vi "Load by Identifier.vi"(8 "error in (no error)":errorcluster, 10 "Identifier":string, 11 "User Provider in":refnum<class "User Provider.lvclass">) -> (0 "error out":errorcluster, 2 "User":refnum<class "User.lvclass">, 3 "User Provider out":refnum<class "User Provider.lvclass">)   [LabVIEW 2022 SP3, in "HTTP-Conditum.lvlib" / "User Provider.lvclass"]
uses:
  User Provider.lvclass
  <vilib>/IlluminatedG/IG HTTP Server/HTTP Server/User/User.lvclass
  User Provider.lvclass/User Provider.ctl
  User/User.lvclass
  <vilib>/IlluminatedG/IG Conditum/Conditum/Columns/String/String.lvclass
  <vilib>/IlluminatedG/IG Conditum/Conditum/Entity Manager/Entity Manager.lvclass
  C:/Program Files (x86)/National Instruments/LabVIEW 2022/vi.lib/IlluminatedG/IG Conditum/Conditum/Entity/Entity.lvclass
  C:/Program Files (x86)/National Instruments/LabVIEW 2022/vi.lib/IlluminatedG/IG HTTP Server/HTTP Server/User/User.lvclass
  C:/Program Files (x86)/National Instruments/LabVIEW 2022/vi.lib/IlluminatedG/IG HTTP Server/HTTP Server/Service/Service.lvclass
  C:/dev/lv/illuminated-g/lv-http-conditum/HTTP-Conditum/User/User.lvclass
  C:/Program Files (x86)/National Instruments/LabVIEW 2022/vi.lib/IlluminatedG/IG Conditum/Conditum/Columns/Type/Type.lvclass
  C:/Program Files (x86)/National Instruments/LabVIEW 2022/vi.lib/IlluminatedG/IG Conditum/Conditum/Columns/String/String.lvclass
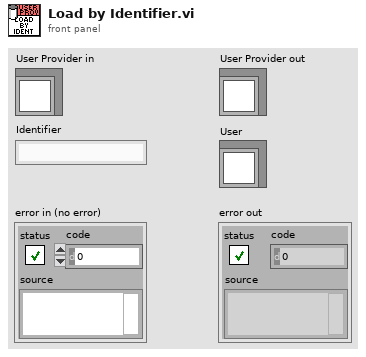
[diagram p1: front panel]
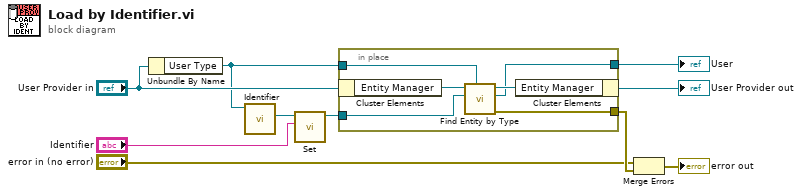
[diagram p0: block diagram]
diagram:
  n1 = Unbundle By Name("User Provider in") -> ("User Type"=w6:refnum<class "User.lvclass">)
  n2 = call "Identifier.vi"("User in"=w6) -> ("Identifier"=w10:refnum<class "String.lvclass">)  [unwired: 10 in]
  n3 = call <vilib>:"Set.vi"("Value"="Identifier", "String in"=w10) -> ("String out"=w8:refnum<class "String.lvclass">)  [unwired: 9 in]
  n4 = in-place {
    in-place-border: w8 -> [w15]
    in-place-border: w6 -> [w14]
    in-place-border: [w12] -> w5
    in-place-border: [w11] -> w3
    n5 = in-place-cluster #1("User Provider in") -> ("Entity Manager"=w16:refnum<class "Entity Manager.lvclass">)
    n6 = call <vilib>:"Find Entity by Type.vi"("Entity Type"=w14, "Type"=w15, "Entity Manager in"=w16) -> ("error out"=w11:errorcluster, "Entity"=w12:refnum<class "User.lvclass">, "Entity Manager out"=w13:refnum<class "Entity Manager.lvclass">)  [unwired: 6 in]
    n7 = in-place-cluster #1("Entity Manager"=w13) -> (→"User Provider out":refnum<class "User Provider.lvclass">)
  }
  "User" <- w5
  n8 = Merge Errors("error in (no error)", w3) -> (→"error out":errorcluster)
